vi "Sting_umwandeln.vi"(0 "Lesepuffer":string, 11 "error in (no error)":errorcluster caption="Fehler (Eingang, kein Fehler)") -> (4 "Device":string, 6 "Zahl 2":dbl, 8 "Zahl 3":dbl, 10 "Gasname":string, 13 "Gase":string, 14 "Array":string[](array[string]), 15 "error out":errorcluster caption="Fehler (Ausgang)")   [LabVIEW 2020, in "Linearisierung v2.lvlib" / "Gasteiler.lvlib" / "HovaCal.lvlib"]
uses:
  HovaCal.lvlib
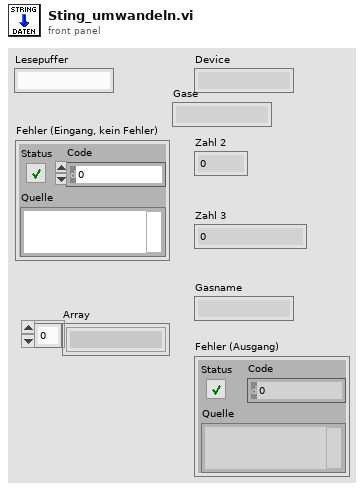
[diagram p1: front panel]
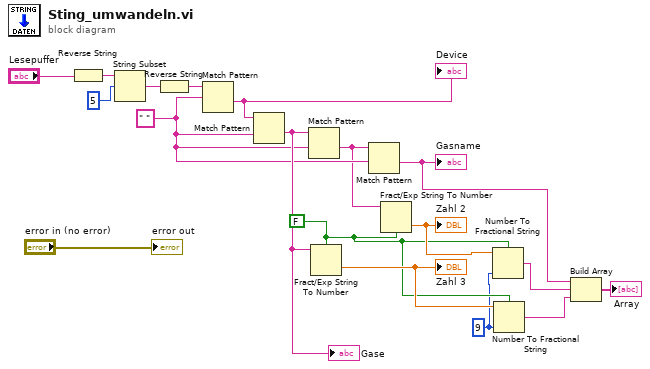
[diagram p0: block diagram]
diagram:
  w1 = i16 9 ("Genauigkeit (6)")
  w2 = FALSE ("Systemdezimalzeichen verwenden (T)")
  w12 = " " ("Nach String/Zeichen suchen (-)")
  n1 = Reverse String(1:"Lesepuffer") -> (0:w10:string)
  n2 = String Subset(string=w10, offset (0)=5 ("Offset (0)")) -> (substring=w15:string)  [unwired: 1 in]
  n3 = Reverse String(1:w15) -> (0:w13:string)
  n4 = Match Pattern(string=w13, regular expression=w12) -> (after substring=w17:string)  [unwired: 1 in, 3 out]
  "Device" <- w17
  n5 = Match Pattern(string=w17, regular expression=w12) -> (after substring=w16:string)  [unwired: 1 in, 3 out]
  "Gase" <- w16
  n6 = Match Pattern(string=w16, regular expression=w12) -> (after substring=w11:string)  [unwired: 1 in, 3 out]
  n7 = Fract/Exp String To Number(use system decimal point (T)=w2, string=w16) -> (number=w7:dbl)  [unwired: 2 in, 1 out]
  "Zahl 3" <- w7
  n8 = Match Pattern(string=w11, regular expression=w12) -> (after substring=w6:string)  [unwired: 1 in, 3 out]
  "Gasname" <- w6
  n9 = Fract/Exp String To Number(use system decimal point (T)=w2, string=w11) -> (number=w8:dbl)  [unwired: 2 in, 1 out]
  "Zahl 2" <- w8
  n10 = Number To Fractional String(use system decimal point (T)=w2, number=w8, precision (6)=w1) -> (F-format string=w5:string)  [unwired: 1 in]
  n11 = Number To Fractional String(use system decimal point (T)=w2, number=w7, precision (6)=w1) -> (F-format string=w4:string)  [unwired: 1 in]
  n12 = Build Array(w6, w5, w4) -> (→"Array":string[])
  "error out" <- "error in (no error)"
